vi "Save GIF Image (Memory).vi"(8 "error in (no error)":errorcluster, 9 "Dither (None)":T1, 10 "Image":T2) -> (0 "error out":errorcluster, 3 "Encoded Image":u8[](array[numeric]))   [LabVIEW 2020, in "G-Image.lvlib"]
doc: "Saves an image in GIF format and returns the encoded image as a byte array..\n\nIf the input image has an alpha channel or mask, it will be used to set the transparent pixels of the resulting GIF image."
uses:
  G-Image.lvlib
  <vilib>/picture/picture.llb/imagedata.ctl
  Controls/Dither Type.ctl
  Controls/Image Save Format.ctl
  9e18263a-0d77-4343-b0c9-39cee55056e0.vi
  Private/Result To Error.vi
  Private/Get Image Data.vi
  Private/ARGB To RGBA.vi
  Private/Depth To Number Channels.vi
  Image Processing/To True Color Image.vi
  <vilib>/Utility/error.llb/Error Cluster From Error Code.vi
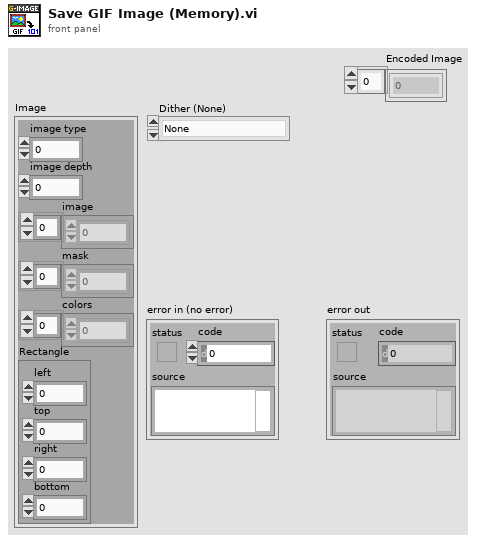
[diagram p1: front panel]
types:
  T1 = typedef "G-Image.lvlib/Dither Type.ctl" = enum32{"None", "Floyd-Steinberg"}
  T2 = typedef "imagedata.ctl" = cluster{"image type":i32, "image depth":i32, "image":u8[], "mask":u8[], "colors":u32[], "Rectangle":cluster{"left":i16, "top":i16, "right":i16, "bottom":i16}}
  T3 = typedef "G-Image.lvlib/Image Save Format.ctl" = enum16{"png", "jpg", "bmp", "gif", "tga", "qoi"}
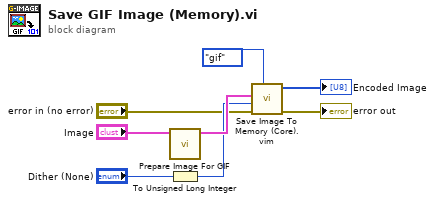
[diagram p0: block diagram]
diagram:
  n1 = call "Prepare Image For GIF.vi"("Image"="Image") -> ("Image"=w5:T2)  [unwired: 9 in, 1 out]
  n2 = To Unsigned Long Integer(number="Dither (None)") -> (unsigned 32bit integer=w4:u32)
  n3 = call "Save Image To Memory (Core).vim"("Save Format"=Image_Save_Format."gif", "error in (no error)"="error in (no error)", "Option"=w4, "Image"=w5) -> ("error out"=→"error out":errorcluster, "Encoded Image"=→"Encoded Image":u8[])  [unwired: 6 in]
